vi "Close VI Server Application Control.vi"(8 "error in (no error)":errorcluster, 11 "VI refnum":refnum<vi>) -> (0 "error out":errorcluster)   [LabVIEW 2011]
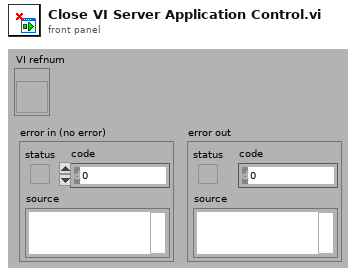
[diagram p1: front panel]
types:
  T1 = enum32{"Bad", "Idle", "Run top level", "Running"}
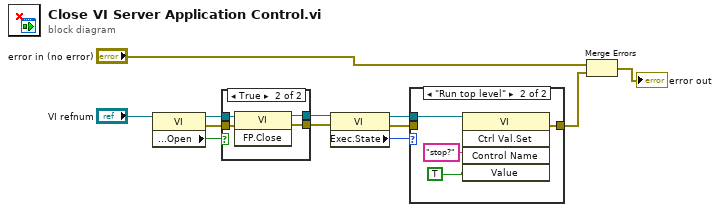
[diagram p0: block diagram]
diagram:
  n1 = property class="VI"(reference="VI refnum") -> (reference out=w11:refnum<vi>, error out=w12:errorcluster, "Front Panel.Open"=w10:bool)  [unwired: 1 in]
  n2 = case shown="True" w10 {
    tunnel: [w14 w18] -> w7
    tunnel: [w13 w17] -> w8
    tunnel: w11 -> [w14 w16]
    tunnel: w12 -> [w13 w15]
    frame False {
    }
    frame True {
      n3 = invoke class="VI" method="FP.Close"(reference=w16, error in=w15) -> (reference out=w18:refnum<vi>, error out=w17:errorcluster)  [unwired: 1 in, 1 out]
    }
  }
  n4 = property class="VI"(reference=w7, error in=w8) -> (reference out=w5:refnum<vi>, error out=w6:errorcluster, "Exec.State"=w4:T1)
  n5 = case shown="\"Run top level\"" w4 {
    tunnel: w5 -> [_ w23]
    tunnel: w6 -> [w19 _]
    tunnel: [w19 w20] -> w2
    frame Default {
    }
    frame "Run top level" {
      n6 = invoke class="VI" method="Ctrl Val.Set"(reference=w23, "Control Name"="stop?", "Value"=TRUE) -> (error out=w20:errorcluster)  [unwired: 2 in, 4 out]
    }
  }
  n7 = Merge Errors("error in (no error)", w2) -> (→"error out":errorcluster)
